vi "Set Robot Position.vi"(5 "Goal":cluster{"X":dbl, "Y":dbl}, 6 "Wheel theta":dbl[](array[numeric])=[200.0, -200.0, -200.0, 200.0], 7 "Odometry Data":dbl[](array[numeric]), 8 "error in (no error)":errorcluster, 9 "axles":refnum<vi>[](array[refnum]), 10 "robot":refnum<vi>, 11 "scene in":refnum<vi>) -> (0 "error out":errorcluster, 3 "scene out":refnum<vi>)   [LabVIEW 2011]
uses:
  <vilib>/picture/3D Picture Control/NI_3D Picture Control.lvlib
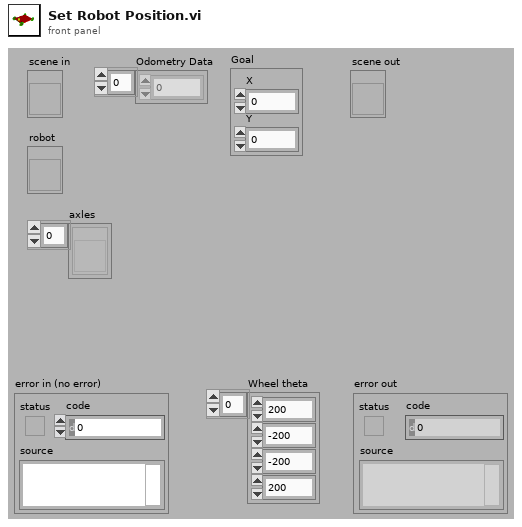
[diagram p1: front panel]
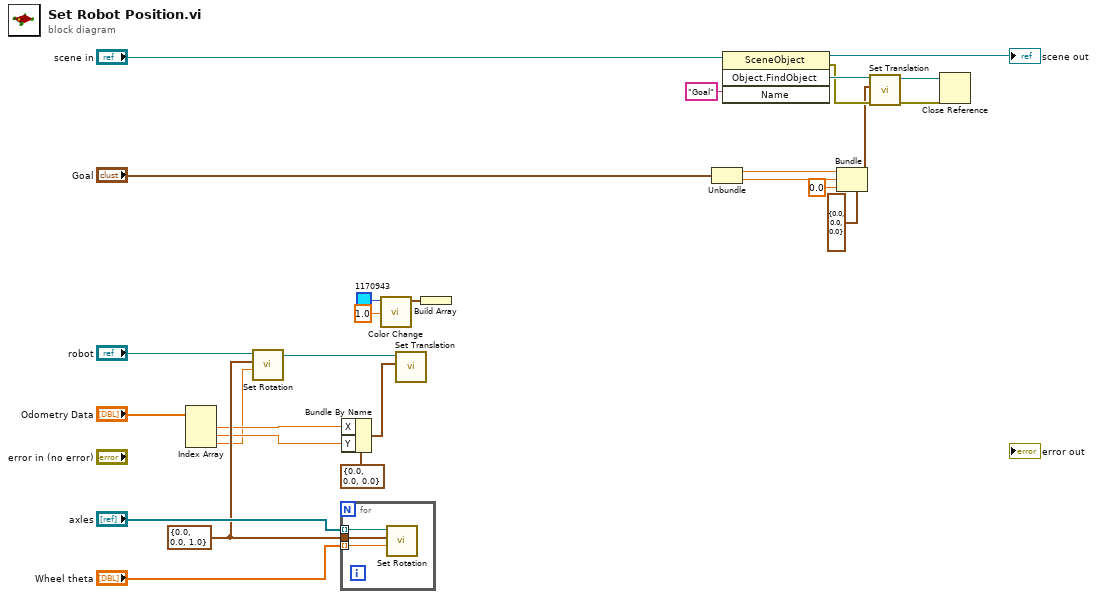
[diagram p0: block diagram]
diagram:
  w24 = cluster{"X":sgl, "Y":sgl, "Z":sgl} {"X"=0.0, "Y"=0.0, "Z"=1.0} ("Axis")
  n1 = Index Array(array="Odometry Data") -> (element #1=w22:dbl, element #2=w21:dbl, element #3=w1:dbl)  [unwired: 3 in]
  n2 = call <vilib>:"Set Rotation.vi"("Angle"=w1, "Axis"=w24, "Scene Object"="robot") -> ("Rotated Scene Object"=w19:refnum<vi>)  [unwired: 1 in, 7 out]
  n3 = for {
    tunnel: "axles" -> [w29] mode=indexing
    tunnel: w24 -> [w30]
    tunnel: "Wheel theta" -> [w28] mode=indexing
    n4 = call <vilib>:"Set Rotation.vi"("Angle"=w28, "Axis"=w30, "Scene Object"=w29) -> ()  [unwired: 1 in, 8 out]
  }
  n5 = Bundle By Name(cluster=cluster{"X":sgl, "Y":sgl, "Z":sgl} {"X"=0.0, "Y"=0.0, "Z"=0.0} ("Axis"), "X"=w22, "Y"=w21) -> (w20:cluster{"X":sgl, "Y":sgl, "Z":sgl})
  n6 = call <vilib>:"Color Change.vi"("Alpha"=1.0, "Color"=u32 1170943) -> ("RGBA"=w15:cluster{"R":sgl, "G":sgl, "B":sgl, "A":sgl})  [unwired: 9 out]
  n7 = call <vilib>:"Set Translation.vi"("Translation"=w20, "Scene Object"=w19) -> ()  [unwired: 1 in, 9 out]
  n8 = Build Array(w15) -> ()  [unwired: 1 out]
  n9 = Unbundle("Goal") -> ("X"=w6:dbl, "Y"=w5:dbl)
  n10 = invoke class="SceneObject" method="Object.FindObject"(reference="scene in", "Name"="Goal") -> (reference out=→"scene out":refnum<vi>, error out=w10:errorcluster, "FindObject"=w12:refnum<vi>)  [unwired: 2 in, 1 out]
  n11 = Bundle(cluster=cluster{"X":sgl, "Y":sgl, "Z":sgl} {"X"=0.0, "Y"=0.0, "Z"=0.0} ("Translation"), "X"=w6, "Y"=w5, "Z"=sgl 0.0) -> (w3:cluster{"X":sgl, "Y":sgl, "Z":sgl})
  n12 = call <vilib>:"Set Translation.vi"("error in (no error)"=w10, "Translation"=w3, "Scene Object"=w12) -> ("error out"=w9:errorcluster, "Translated Object"=w11:refnum<vi>)  [unwired: 7 out]
  n13 = Close Reference(reference=w11, error in (no error)=w9) -> ()  [unwired: 1 out]
